vi "ADO Connection Set Timeout.vi"(8 "error in (no error)":errorcluster, 10 "ConnectionTimeout":i32, 11 "ADODB._Connection":refnum<k7>) -> (0 "error out":errorcluster, 3 "ADODB._Connection":refnum<k7>)   [LabVIEW 2013]
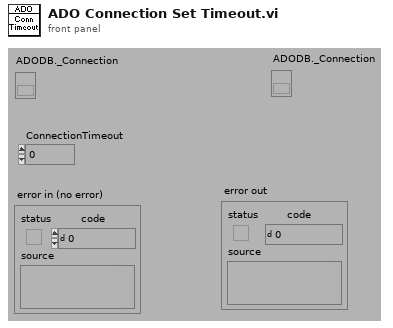
[diagram p1: front panel]
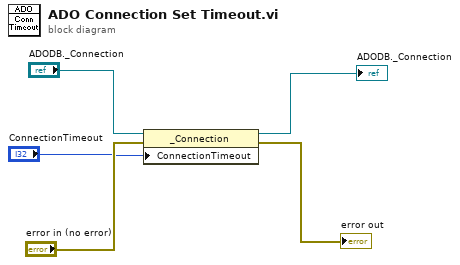
[diagram p0: block diagram]
diagram:
  n1 = property class="_Connection"(reference="ADODB._Connection", error in="error in (no error)", "ConnectionTimeout"="ConnectionTimeout") -> (reference out=→"ADODB._Connection":refnum<k7>, error out=→"error out":errorcluster)
